vi "Upload Part.vi"(4 "Region":T1, 7 "Content MD5":string, 8 "error in (no error)":errorcluster, 9 "Part Number":u16=1 min=1 max=10000, 10 "Data":string, 11 "Multipart Upload RefNum in":T2) -> (0 "error out":errorcluster, 2 "Success?":bool, 3 "Multipart Upload RefNum out":T2)   [LabVIEW 2015, in "LV Interface for Amazon S3.lvlib"]
doc: "This operation <B>uploads a part in a multipart upload</B>. <B>You must initiate a multipart upload</B> (see Initiate Multipart Upload.vi) <B>before you can upload any part</B>. In response to your initiate request, you will receive a Multipart Upload Refnum, that you must use through the whole upload process."
uses:
  LV Interface for Amazon S3.lvlib
  Typedefs/AMZ_S3_Multipart Upload RefNum.ctl
  Typedefs/AMZ_S3_Multipart Upload RefNum Enum.ctl
  Typedefs/AMZ_S3_LocationConstraint.ctl
  Typedefs/AMZ_S3_HTTP Header-Value pair.ctl
  Typedefs/AMZ_S3_Multipart Upload Part Data.ctl
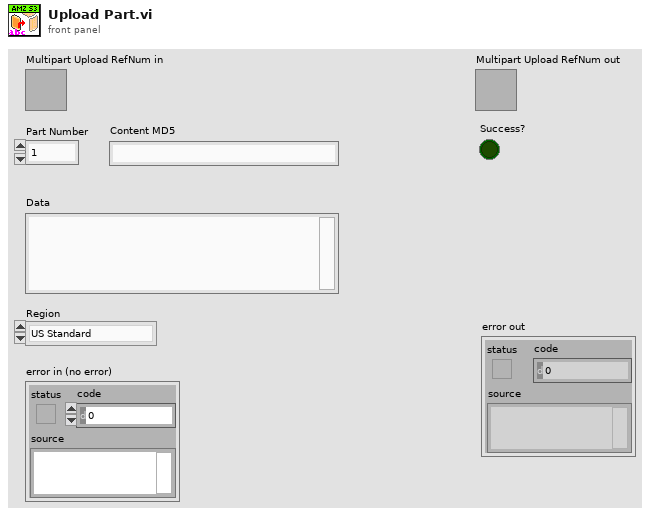
[diagram p1: front panel]
types:
  T1 = typedef "LV Interface for Amazon S3.lvlib/AMZ_S3_LocationConstraint.ctl" = enum16{"US Standard", "us-east-2", "us-west-1", "us-west-2", "ap-northeast-1", "ap-northeast-2", "ap-southeast-1", "ap-southeast-2", "ca-central-1", "eu-central-1", "eu-west-1", "eu-west-2", "sa-east-1"}
  T2 = typedef "LV Interface for Amazon S3.lvlib/AMZ_S3_Multipart Upload RefNum.ctl" = refnum<k1>
  T3 = typedef "LV Interface for Amazon S3.lvlib/AMZ_S3_Multipart Upload Data.ctl" = cluster{"Object":string, "Bucket":string, "UploadID":string, "Parts":T4[]}
  T4 = typedef "LV Interface for Amazon S3.lvlib/AMZ_S3_Multipart Upload Part Data.ctl" = cluster{"PartNumber":u16, "Lat modified":timestamp, "ETag":string, "Size":u64}
  T5 = typedef "LV Interface for Amazon S3.lvlib/AMZ_S3_HTTP Header-Value pair.ctl" = cluster{"Header":string, "Value":string}
  T6 = cluster{"format string":string, "UploadID":string}
  T7 = cluster{"format string":string, "UploadID":string}[]
  T8 = typedef "LV Interface for Amazon S3.lvlib/AMZ_S3_Call Results.ctl" = enum16{"Success", "UndefinedError", "AccessDenied", "AccountProblem", "AmbiguousGrantByEmailAddress", "BadDigest", "BucketAlreadyExists", "BucketAlreadyOwnedByYou", "BucketNotEmpty", "CredentialsNotSupported", "CrossLocationLoggingProhibited", "EntityTooSmall", "EntityTooLarge", "ExpiredToken", "IllegalVersioningConfigurationException", "IncompleteBody", "IncorrectNumberOfFilesInPostRequest", "InlineDataTooLarge", "InternalError", "InvalidAccessKeyId", "InvalidAddressingHeader", "InvalidArgument", "InvalidBucketName", "InvalidDigest", "InvalidLocationConstraint", "InvalidPart", "InvalidPartOrder", "InvalidPayer", "InvalidPolicyDocument", "InvalidRange", "InvalidSecurity", "InvalidSOAPRequest", "InvalidStorageClass", "InvalidTargetBucketForLogging", "InvalidToken", "InvalidURI", "KeyTooLong", "MalformedACLError", "MalformedPOSTRequest", "MalformedXML", "MaxMessageLengthExceeded", "MaxPostPreDataLengthExceededError", "MetadataTooLarge", "MethodNotAllowed", "MissingAttachment", "MissingContentLength", "MissingRequestBodyError", "MissingSecurityElement", "MissingSecurityHeader", "NoLoggingStatusForKey", "NoSuchBucket", "NoSuchKey", "NoSuchUpload", "NoSuchVersion", "NotImplemented", "NotSignedUp", "OperationAborted", "PermanentRedirect", "PreconditionFailed", "Redirect", "RequestIsNotMultiPartContent", "RequestTimeout", "RequestTimeTooSkewed", "RequestTorrentOfBucketError", "SignatureDoesNotMatch", "SlowDown", "TemporaryRedirect", "TokenRefreshRequired", "TooManyBuckets", "UnexpectedContent", "UnresolvableGrantByEmailAddress", "UserKeyMustBeSpecified", "LabVIEWError"}
  T9 = typedef "LV Interface for Amazon S3.lvlib/AMZ_S3_API_UploadPartResult.ctl" = cluster{"ETag":string}
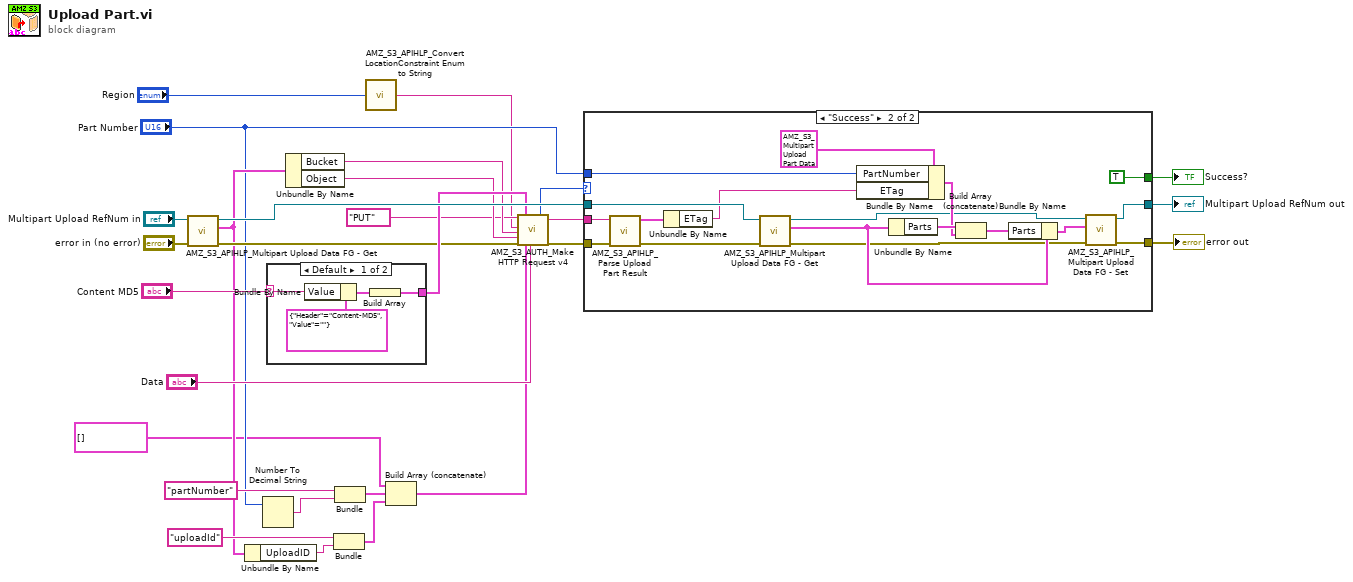
[diagram p0: block diagram]
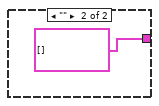
[diagram p2: hidden frame]
diagram:
  n1 = call "AMZ_S3_APIHLP_Multipart Upload Data FG - Get.vi"("error in (no error)"="error in (no error)", "Multipart Upload RefNum in"="Multipart Upload RefNum in") -> ("error out"=w14:errorcluster, "Multipart Upload Data"=w10:T3, "Multipart Upload RefNum out"=w22:T2)  [unwired: 7 in]
  n2 = Unbundle By Name(w10) -> ("UploadID"=w9:string)
  n3 = Number To Decimal String(number="Part Number") -> (decimal integer string=w7:string)  [unwired: 1 in]
  n4 = case shown="Default" "Content MD5" {
    selector: "Content MD5" -> [w30 _]
    tunnel: [w29 T5[] []] -> w20
    frame Default {
      n5 = Bundle By Name(cluster=T5 {"Header"="Content-MD5", "Value"=""} ("HTTP Header-Value pair"), "Value"=w30) -> (w32:T5)
      n6 = Build Array(w32) -> (w29:T5[])
    }
    frame "" {
    }
  }
  n7 = Unbundle By Name(w10) -> ("Bucket"=w16:string, "Object"=w15:string)
  n8 = Bundle("format string"="uploadId", "UploadID"=w9) -> (w4:T6)  [unwired: 1 in]
  n9 = Bundle("format string"="partNumber", w7) -> (w5:cluster{"format string":string, string})  [unwired: 1 in]
  n10 = call "AMZ_S3_APIHLP_Convert LocationConstraint Enum to String.vi"("Location"="Region") -> ("Location String"=w1:string)  [unwired: 4 in]
  n11 = Build Array (concatenate)(cluster{"item":string, "value":string}[] [] ("request parameters"), w5, w4) -> (w3:T7)
  n12 = call "AMZ_S3_AUTH_Make HTTP Request v4.vi"("HTTP-Verb"="PUT", "Region"=w1, "Bucket"=w16, "Object Key"=w15, "error in"=w14, "request headers"=w20, "request parameters"=w3, "request body"="Data") -> ("Call Result"=w19:T8, "response headers"=w18:string, "error out"=w17:errorcluster)  [unwired: 8 in, 1 out]
  n13 = case shown="\"Success\"" w19 {
    tunnel: w17 -> [w34 w53]
    tunnel: w22 -> [w35 w49]
    tunnel: [w35 w38] -> w27
    tunnel: w18 -> [_ w52]
    tunnel: "Part Number" -> [_ w46]
    tunnel: [w34 w37] -> w25
    tunnel: [_ TRUE] -> w26
    frame Default {
    }
    frame "Success" {
      n14 = call "AMZ_S3_APIHLP_Parse Upload Part Result.vi"("error in (no error)"=w53, "Response header"=w52) -> ("error out"=w50:errorcluster, "UploadPartResult"=w51:T9)  [unwired: 8 in]
      n15 = Unbundle By Name(w51) -> ("ETag"=w45:string)
      n16 = call "AMZ_S3_APIHLP_Multipart Upload Data FG - Get.vi"("error in (no error)"=w50, "Multipart Upload RefNum in"=w49) -> ("error out"=w39:errorcluster, "Multipart Upload Data"=w42:T3, "Multipart Upload RefNum out"=w43:T2)  [unwired: 7 in]
      n17 = Bundle By Name(cluster=T4 {"PartNumber"=0, "Lat modified"=timestamp(0 s since 1904-01-01), "ETag"="", "Size"=0} ("Multipart Upload Part"), "PartNumber"=w46, "ETag"=w45) -> (w44:T4)
      n18 = Unbundle By Name(w42) -> ("Parts"=w48:T4[])
      n19 = Build Array (concatenate)(w48, w44) -> (w41:T4[])
      n20 = Bundle By Name(cluster=w42, "Parts"=w41) -> (w40:T3)
      n21 = call "AMZ_S3_APIHLP_Multipart Upload Data FG - Set.vi"("error in (no error)"=w39, "Multipart Upload Data"=w40, "Multipart Upload RefNum in"=w43) -> ("error out"=w37:errorcluster, "Multipart Upload RefNum out"=w38:T2)  [unwired: 6 in, 1 out]
    }
  }
  "Multipart Upload RefNum out" <- w27
  "Success?" <- w26
  "error out" <- w25
